vi "试剂余量后台任务.vi"   [LabVIEW 2016, in "斯坦道氨氮.lvlib"]
uses:
  <vilib>/ptbypt/NI_PtbyPt.lvlib
types:
  T1 = cluster{"V1":sgl, "V2":sgl, "V3":sgl, "V4":sgl, "V5":sgl, "V6":sgl, "V7":sgl, "V8":sgl, "V9":sgl, "V10":sgl, "V11":sgl, "V12":sgl, "V9-1":sgl, "V9-2":sgl}
  T2 = typedef "报警信息字段定义.ctl" = cluster{"时间":timestamp, "参数":string, "报警信息":string, "备注":string, "code":u64}
  T3 = cluster{"系统时间":timestamp, "工作状态":u16, "测量模式":enum16{"待机", "连续模式", "周期模式", "定点模式", "受控模式", "手动模式"}, "告警代码":u16, "故障代码":u16, "日志代码":u16, "软件版本":u16, "F0":sgl, "F1":sgl, "F2":sgl, "F3":sgl, "T":sgl, "H":sgl, "id":u16, "flowid":u16, "量程":u16, "总磷控温温度1":sgl, "营养盐控温温度2":sgl, "ADC":sgl}
  T4 = cluster{"V1":bool, "V2":bool, "V3":bool, "V4":bool, "V5":bool, "V6":bool, "V7":bool, "V8":bool, "V9":bool, "V10":bool, "V11":bool, "V12":bool, "V9-1":bool, "V9-2":bool}
  T5 = cluster{"参数":string, "报警内容":string, "报警分析":string}
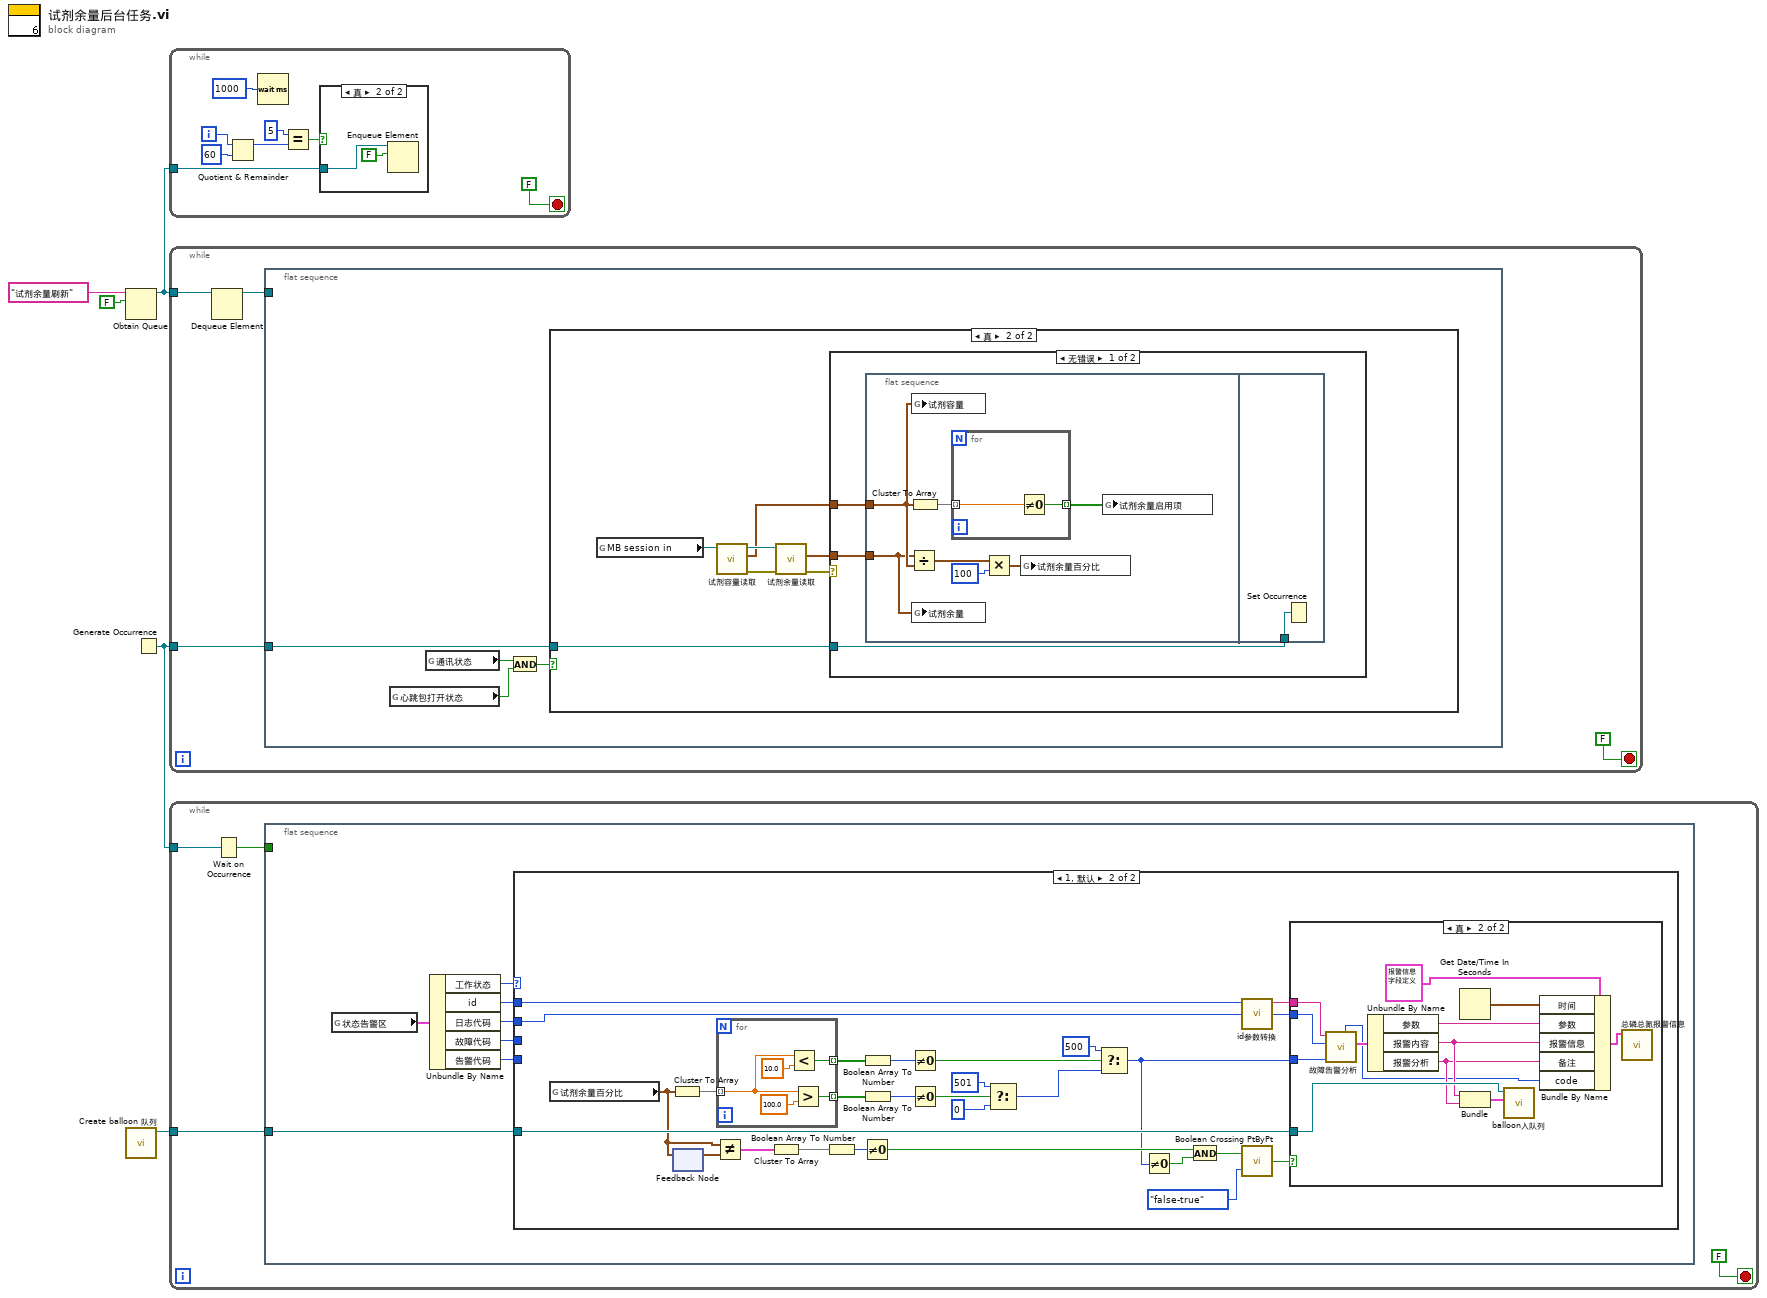
[diagram p0: block diagram]
diagram:
  n1 = Obtain Queue(name (unnamed)="试剂余量刷新" ("名称（未命名）"), element data type=FALSE) -> (queue out=w1:refnum<queue>)  [unwired: 3 in, 2 out]
  n2 = call "Create balloon 队列.vi"() -> ("队列输出"=w5:refnum<queue>)  [unwired: 11 in]
  n3 = Generate Occurrence() -> (w4:refnum<k4>)
  n4 = while {
    tunnel: w1 -> [w12]
    i -> [w10]
    stop <- FALSE stop-if-true
    n5 = Quotient & Remainder(x=w10, y=60) -> (x-y*floor(x/y)=w8:i32)  [unwired: 1 out]
    n6 = Wait (ms)(milliseconds to wait=u32 1000 ("等待时间（毫秒）")) -> ()  [unwired: 1 out]
    n7 = Equal?(x=5, y=w8) -> (x = y?=w7:bool)
    n8 = case shown="真" w7 {
      tunnel: w12 -> [_ w15]
      frame False {
      }
      frame True {
        n9 = Enqueue Element(queue=w15, element=FALSE ("元素")) -> ()  [unwired: 2 in, 3 out]
      }
    }
  }
  n10 = while {
    tunnel: w4 -> [w18]
    tunnel: w1 -> [w17]
    stop <- FALSE stop-if-true
    n11 = Dequeue Element(queue=w17) -> (queue out=w16:refnum<queue>)  [unwired: 2 in, 3 out]
    n12 = flat-sequence {
      tunnel: w18 -> [w23]
      tunnel: w16 -> [_]
      frame #0 {
        n13 = global read "VAR总磷总氮全局变量.vi" "心跳包打开状态"() -> (w22:bool)
        n14 = global read "VAR总磷总氮全局变量.vi" "通讯状态"() -> (w20:bool)
        n15 = And(x=w20, y=w22) -> (x .and. y?=w21:bool)
        n16 = case shown="真" w21 {
          tunnel: w23 -> [_ w24]
          frame False {
          }
          frame True {
            n17 = global read "VAR总磷总氮全局变量.vi" "MB session in"() -> (w28:refnum<class "MB_Master.lvclass">)
            n18 = call "试剂容量读取.vi"("MB session in"=w28) -> ("error out"=w30:errorcluster, "试剂容量"=w27:T1, "MB session out"=w29:refnum<class "MB_Master.lvclass">)  [unwired: 8 in]
            n19 = call "试剂余量读取.vi"("Error in"=w30, "MB session in"=w29) -> ("error out"=w25:errorcluster, "试剂余量"=w26:T1)  [unwired: 7 in, 1 out]
            n20 = case shown="无错误" w25 {
              tunnel: w27 -> [w33 _]
              tunnel: w26 -> [w32 _]
              tunnel: w24 -> [w31 _]
              frame No Error {
                n21 = flat-sequence {
                  tunnel: w33 -> [w38]
                  tunnel: w32 -> [w37]
                  tunnel: w31 -> [w43]
                  frame #0 {
                    n22 = Divide(x=w37, y=w38) -> (x/y=w40:T1)
                    n23 = Cluster To Array(cluster=w38) -> (array=w35:sgl[])
                    n24 = global write "VAR总磷总氮全局变量.vi" "试剂容量"(w38) -> ()
                    n25 = global write "VAR总磷总氮全局变量.vi" "试剂余量"(w37) -> ()
                    n26 = for {
                      tunnel: w35 -> [w42] mode=indexing
                      tunnel: [w41] -> w34 mode=indexing
                      n27 = Not Equal To 0?(x=w42) -> (x != 0?=w41:bool)
                    }
                    n28 = Multiply(x=w40, y=100) -> (x*y=w36:T1)
                    n29 = global write "VAR总磷总氮全局变量.vi" "试剂余量百分比"(w36) -> ()
                    n30 = global write "VAR总磷总氮全局变量.vi" "试剂余量启用项"(w34) -> ()
                  }
                  frame #1 {
                    n31 = Set Occurrence(w43) -> ()
                  }
                }
              }
              frame Error {
              }
            }
          }
        }
      }
    }
  }
  n32 = while {
    tunnel: w5 -> [w46]
    tunnel: w4 -> [w45]
    stop <- FALSE stop-if-true
    n33 = Wait on Occurrence(2:w45) -> (0:w44:bool)  [unwired: 2 in]
    n34 = flat-sequence {
      tunnel: w46 -> [w52]
      tunnel: w44 -> [_]
      frame #0 {
        n35 = global read "VAR总磷总氮全局变量.vi" "状态告警区"() -> (w48:T3)
        n36 = Unbundle By Name(w48) -> ("工作状态"=w49:u16, "id"=w54:u16, "日志代码"=w53:u16, "故障代码"=w51:u16, "告警代码"=w50:u16)
        n37 = case shown="1, 默认" w49 {
          tunnel: w54 -> [_ w80]
          tunnel: w53 -> [_ w55]
          tunnel: w52 -> [_ w79]
          tunnel: w51 -> [_ _]
          tunnel: w50 -> [_ _]
          frame 0 {
          }
          frame 1, Default {
            n38 = global read "VAR总磷总氮全局变量.vi" "试剂余量百分比"() -> (w65:T1)
            n39 = Cluster To Array(cluster=w65) -> (array=w74:sgl[])
            n40 = feedback-in #1(w65) -> ()
            n41 = feedback #1() -> (w66:T1)  [unwired: 1 in]
            n42 = Not Equal?(x=w65, y=w66) -> (x != y?=w64:T4)
            n43 = for {
              tunnel: w74 -> [w83] mode=indexing
              tunnel: [w84] -> w76 mode=indexing
              tunnel: [w81] -> w75 mode=indexing
              n44 = Less?(x=w83, y=sgl 10.0) -> (x < y?=w84:bool)
              n45 = Greater?(x=w83, y=sgl 100.0) -> (0:w81:bool)
            }
            n46 = Cluster To Array(cluster=w64) -> (array=w63:bool[])
            n47 = Boolean Array To Number(Boolean array=w63) -> (number=w62:u32)
            n48 = Not Equal To 0?(x=w62) -> (x != 0?=w60:bool)
            n49 = Boolean Array To Number(Boolean array=w76) -> (number=w78:u32)
            n50 = Boolean Array To Number(Boolean array=w75) -> (number=w77:u32)
            n51 = Not Equal To 0?(x=w78) -> (x != 0?=w73:bool)
            n52 = Not Equal To 0?(x=w77) -> (x != 0?=w71:bool)
            n53 = Select(t=501, s=w71, f=0) -> (s? t:f=w68:i32)
            n54 = Select(t=500, s=w73, f=w68) -> (s? t:f=w57:i32)
            n55 = Not Equal To 0?(x=w57) -> (x != 0?=w67:bool)
            n56 = And(x=w60, y=w67) -> (x .and. y?=w61:bool)
            n57 = call "id参数转换.vi"("id"=w80) -> ("table输出"=w56:string)  [unwired: 9 in, 1 out]
            n58 = call <vilib>:"Boolean Crossing PtByPt.vi"("direction"=enum16{"either", "false-true", "true-false"}."false-true", "input"=w61) -> ("crossing"=w59:bool)  [unwired: 1 in]
            n59 = case shown="真" w59 {
              tunnel: w79 -> [_ w98]
              tunnel: w57 -> [_ w91]
              tunnel: w56 -> [_ w89]
              tunnel: w55 -> [_ w88]
              frame False {
              }
              frame True {
                n60 = call "故障告警分析.vi"("告警代码"=w91, "运行步序"=w88, "参数"=w89) -> ("报警内容"=w90:T5, "sysid"=w86:i32)  [unwired: 5 in, 2 out]
                n61 = Unbundle By Name(w90) -> ("参数"=w95:string, "报警内容"=w94:string, "报警分析"=w93:string)
                n62 = Get Date/Time In Seconds() -> (seconds since 1Jan1904=w97:timestamp)
                n63 = Bundle("报警内容"=w94, "报警分析"=w93) -> (w92:cluster{"报警内容":string, "报警分析":string})  [unwired: 1 in]
                n64 = call "balloon入队列.vi"("报警内容"=w92, "队列"=w98) -> ()  [unwired: 9 in, 1 out]
                n65 = Bundle By Name(cluster=T2 {"时间"=timestamp(0 s since 1904-01-01), "参数"="", "报警信息"="", "备注"="", "code"=0} ("data in"), "时间"=w97, "参数"=w95, "报警信息"=w94, "备注"=w93, "code"=w86) -> (w96:T2)
                n66 = call "总磷总氮报警信息.vi"("data in"=w96) -> ()  [unwired: 10 in, 1 out]
              }
            }
          }
        }
      }
    }
  }
